vi "Get Switch Button from Map.vi"(8 "error in (no error)":errorcluster, 10 "Subview Command":string, 11 "URL Refnum Map":variant) -> (0 "error out":errorcluster, 1 "Found?":bool, 2 "Switch Button Refnum":refnum<vi>, 3 "dup URL Refnum Map":variant)   [LabVIEW 2024]
doc: "Gets the switch button refnum from the map."
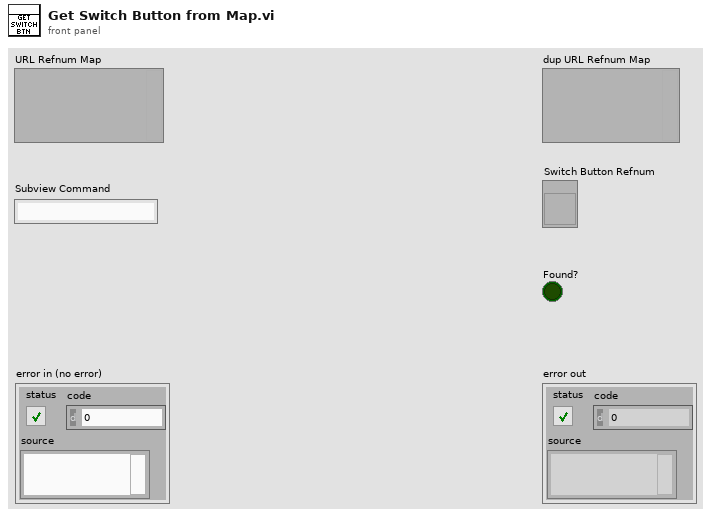
[diagram p1: front panel]
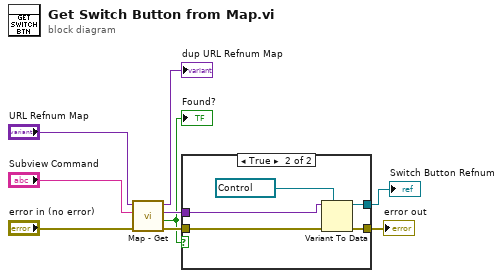
[diagram p0: block diagram]
diagram:
  n1 = call "Map - Get.vi"("error in (no error)"="error in (no error)", "Key"="Subview Command", "Map In"="URL Refnum Map") -> ("error out"=w5:errorcluster, "Found?"=w2:bool, "Value"=w3:variant, "Map Out"=→"dup URL Refnum Map":variant)  [unwired: 5 in]
  "Found?" <- w2
  n2 = case shown="True" w2 {
    tunnel: w5 -> [w10 w15]
    tunnel: [w10 w14] -> w4
    tunnel: w3 -> [_ w13]
    tunnel: [_ w12] -> w1
    frame False {
    }
    frame True {
      n3 = Variant To Data(error in=w15, type=refnum<vi> refnum ("Description"), Variant=w13) -> (data=w12:refnum<vi>, error out=w14:errorcluster)
    }
  }
  "error out" <- w4
  "Switch Button Refnum" <- w1
